vi "test-call.vi"() -> ()   [LabVIEW 2020, in "G-Embedded-Python-Interpreter-Toolkit.lvlib"]
uses:
  G-Embedded-Python-Interpreter-Toolkit/G-Embedded-Python-Interpreter-Toolkit.lvlib
  G-Embedded-Python-Interpreter-Toolkit/Python Object Reference.ctl
  G-Embedded-Python-Interpreter-Toolkit/Python Object Type.ctl
  <vilib>/Utility/error.llb/Error Cluster From Error Code.vi
  <vilib>/ErrorRing/Error Ring.xnode
  <vilib>/Utility/Data Type/NI_Data Type.lvlib
  bin/gepit.cp310.32.dll
panel:
  out "error out 2":errorcluster
  in  "error in (no error) 2":errorcluster
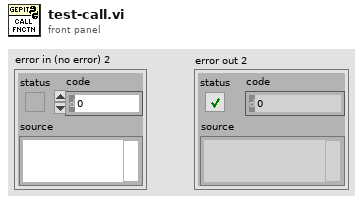
[diagram p1: front panel]
types:
  T1 = typedef "NI_Data Type.lvlib/Data Type.ctl" = enum8{"Invalid Type", "Void", "I8", "I16", "I32", "I64", "U8", "U16", "U32", "U64", "Single Float", "Double Float", "Extended Float", "Single Complex", "Double Complex", "Extended Complex", "Enum U8", "Enum U16", "Enum U32", "Enum U64", "Single Float With Unit", "Double Float With Unit", "Extended Float With Unit", "Single Complex with Unit", "Double Complex with Unit", "Extended Complex with Unit", "Boolean", "String", "Path", "Picture", "Tag", "Array", "Cluster", "Variant", "LV Variant", "Waveform", "Timestamp", "Digital Waveform", "Digital Data", "ExpressData", "Refnum", "External Data", "VI", "Poly VI", "LabVIEW Class Instance", "Fixed Point", "Set Collection", "Map Collection"}
  T2 = typedef "G-Embedded-Python-Interpreter-Toolkit.lvlib/Python Object Reference.ctl" = refnum<k1>
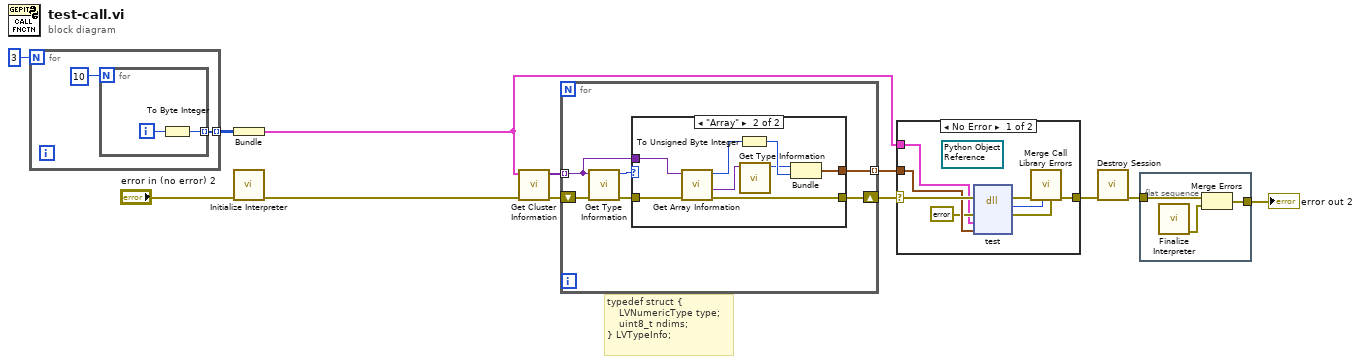
[diagram p0: block diagram]
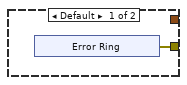
[diagram p2: hidden frame]
diagram:
  # "typedef struct {\n    LVNumericType type;\n    uint8_t ndims;\n} LVTypeInfo;"
  n1 = for {
    N: 3 -> [_]
    tunnel: [w13] -> w9 mode=indexing
    n2 = for {
      N: 10 -> [_]
      tunnel: [w15] -> w13 mode=indexing
      i -> [w16]
      n3 = To Byte Integer(number=w16) -> (8bit integer=w15:i8)
    }
  }
  n4 = Bundle(w9) -> (w2:cluster{i8[][]})  [unwired: 1 in]
  n5 = call "Initialize Interpreter.vi"("error in (no error)"="error in (no error) 2") -> ("error out"=w3:errorcluster)  [unwired: 9 in, 1 out]
  n6 = call <vilib>:"Get Cluster Information.vi"("error in (no error)"=w3, "variant"=w2) -> ("error out"=w7:errorcluster, "cluster elements"=w8:variant[])  [unwired: 8 in]
  n7 = for {
    tunnel: w8 -> [w21] mode=indexing
    tunnel: [w20] -> w6 mode=indexing
    shift-right: [w17] -> w5
    shift-left: w7 -> [w19]
    n8 = call <vilib>:"Get Type Information.vi"("error in (no error)"=w19, "variant"=w21) -> ("error out"=w18:errorcluster, "type"=w22:T1)  [unwired: 5 in, 3 out]
    n9 = case shown="\"Array\"" w22 {
      tunnel: w21 -> [_ w36]
      tunnel: [_ w33] -> w20
      tunnel: w18 -> [_ w32]
      tunnel: [w23 w31] -> w17
      frame Default {
        n10 = xnode "Error Ring"() -> ("error out"=w23:errorcluster)
      }
      frame "Array" {
        n11 = call <vilib>:"Get Array Information.vi"("error in (no error)"=w32, "variant"=w36) -> ("error out"=w31:errorcluster, "array element data type"=w30:variant, "number of dimensions"=w35:i32)  [unwired: 6 in, 1 out]
        n12 = To Unsigned Byte Integer(number=w35) -> (unsigned 8bit integer=w34:u8)
        n13 = call <vilib>:"Get Type Information.vi"("variant"=w30) -> ("type"=w29:T1)  [unwired: 6 in, 4 out]
        n14 = Bundle("type"=w29, w34) -> (w33:cluster{"type":T1, u8})  [unwired: 1 in]
      }
    }
  }
  n15 = case shown="No Error" w5 {
    selector: w5 -> [w44 w45]
    tunnel: [w43 w45] -> w10
    tunnel: w6 -> [w42 _]
    tunnel: w2 -> [w37 _]
    frame No Error {
      (unwired) T2 refnum items=["PObj"] ("Returned Python Object Refnum")
      n16 = dll-call lib="C:/serenial/libraries/g-embedded-python-interpreter-toolkit/LabVIEW/bin/gepit.cp310.32.dll" fn="test"(error in=w44, "Error"=errorcluster {"status"=FALSE, "code"=0, "source"=""} ("error constant"), "Arguments"=w37, "Argument Info"=w42) -> (error out=w40:errorcluster, "return type"=w39:i32, "Error"=w38:errorcluster)  [unwired: 4 in, 1 out]
      n17 = call "Merge Call Library Errors.vi"("Call Library Error"=w38, "Return Value"=w39, "error in"=w40) -> ("error out"=w43:errorcluster)  [unwired: 8 in]
    }
    frame Error {
    }
  }
  n18 = call "Destroy Session.vi"("error in (no error)"=w10) -> ("error out"=w11:errorcluster)  [unwired: 10 in]
  n19 = flat-sequence {
    tunnel: w11 -> [w48]
    tunnel: [w46] -> w12
    frame #0 {
      n20 = call "Finalize Interpreter.vi"() -> ("error out"=w47:errorcluster)  [unwired: 11 in]
      n21 = Merge Errors(w48, w47) -> (w46:errorcluster)
    }
  }
  "error out 2" <- w12
